vi "Test Sequence.vi"(0 "FeedBack Channel":string[](array[string])=["fgdgfvcbc", "vnfhgjkn", "21354682"], 1 "Test Name":string, 2 "Steps":T1(array[cluster]), 4 "WFGraph Refnum":refnum<vi>) -> (6 "Emergency":bool, 7 "Out":i32, 8 "Condition":bool)   [LabVIEW 2015]
uses:
  Galobal variable_TI.vi
  Project Setup/Globle Variable/GR_Servo.vi
  <vilib>/Instr/_visa.llb/VISA Configure Serial Port (Instr).vi
panel:
  out "error out 3":errorcluster
  out "Wait/Poll (ms)":u32
  out "Channels (Out)":i32[](array[numeric])
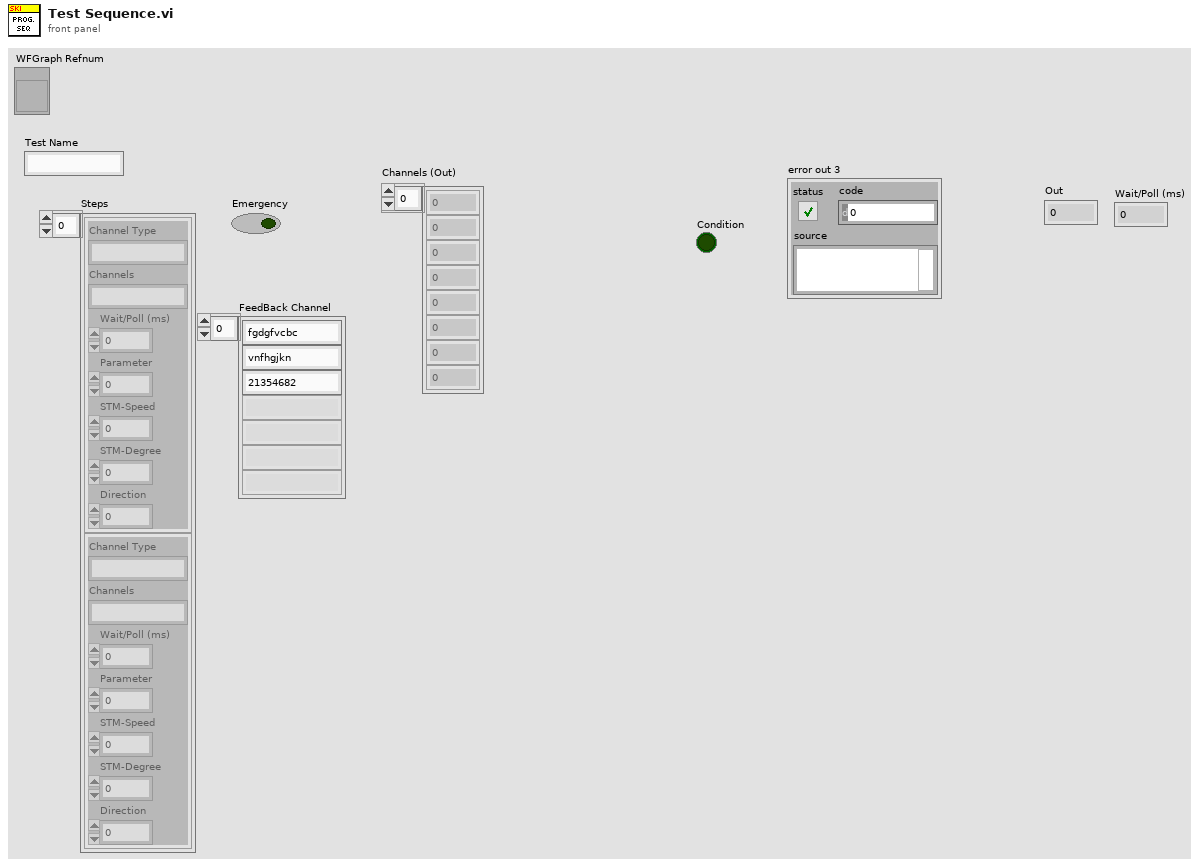
[diagram p1: front panel]
types:
  T1 = cluster{"Channel Type":string, "Channels":string, "Wait/Poll (ms)":u32, "Parameter":u8, "STM-Speed":i32, "STM-Degree":u32, "Direction":u8}[]
  T2 = cluster{"Emergency_1":bool, "Reset_2":bool, "Home _3":bool, "Air Pressure_4":bool, "Safety Sensor_5":bool, "Safety Sensor_6":bool, "Slide Servo Home RS 26":bool, "LVDT UP RS":bool, "Servo Fault 27":bool, "Pressing UP RS 31":bool, "40 Deg. Down Fixture Rs":bool}
  T3 = cluster{"MIC ":refnum<visa-resource-name>, "baud rate MIC ":u32, "LCD ":refnum<visa-resource-name>, "baud rate_LCD":u32}
  T4 = cluster{"Load Max(N)":dbl, "Load Min(N)":dbl, "Actuator1 max(mm)":dbl, "Actuator1min(mm)":dbl, "Actuator2 max(mm)":dbl, "Actuator2min(mm)":dbl, "Load Offset":dbl, "Model":string, "MIC Code":string}
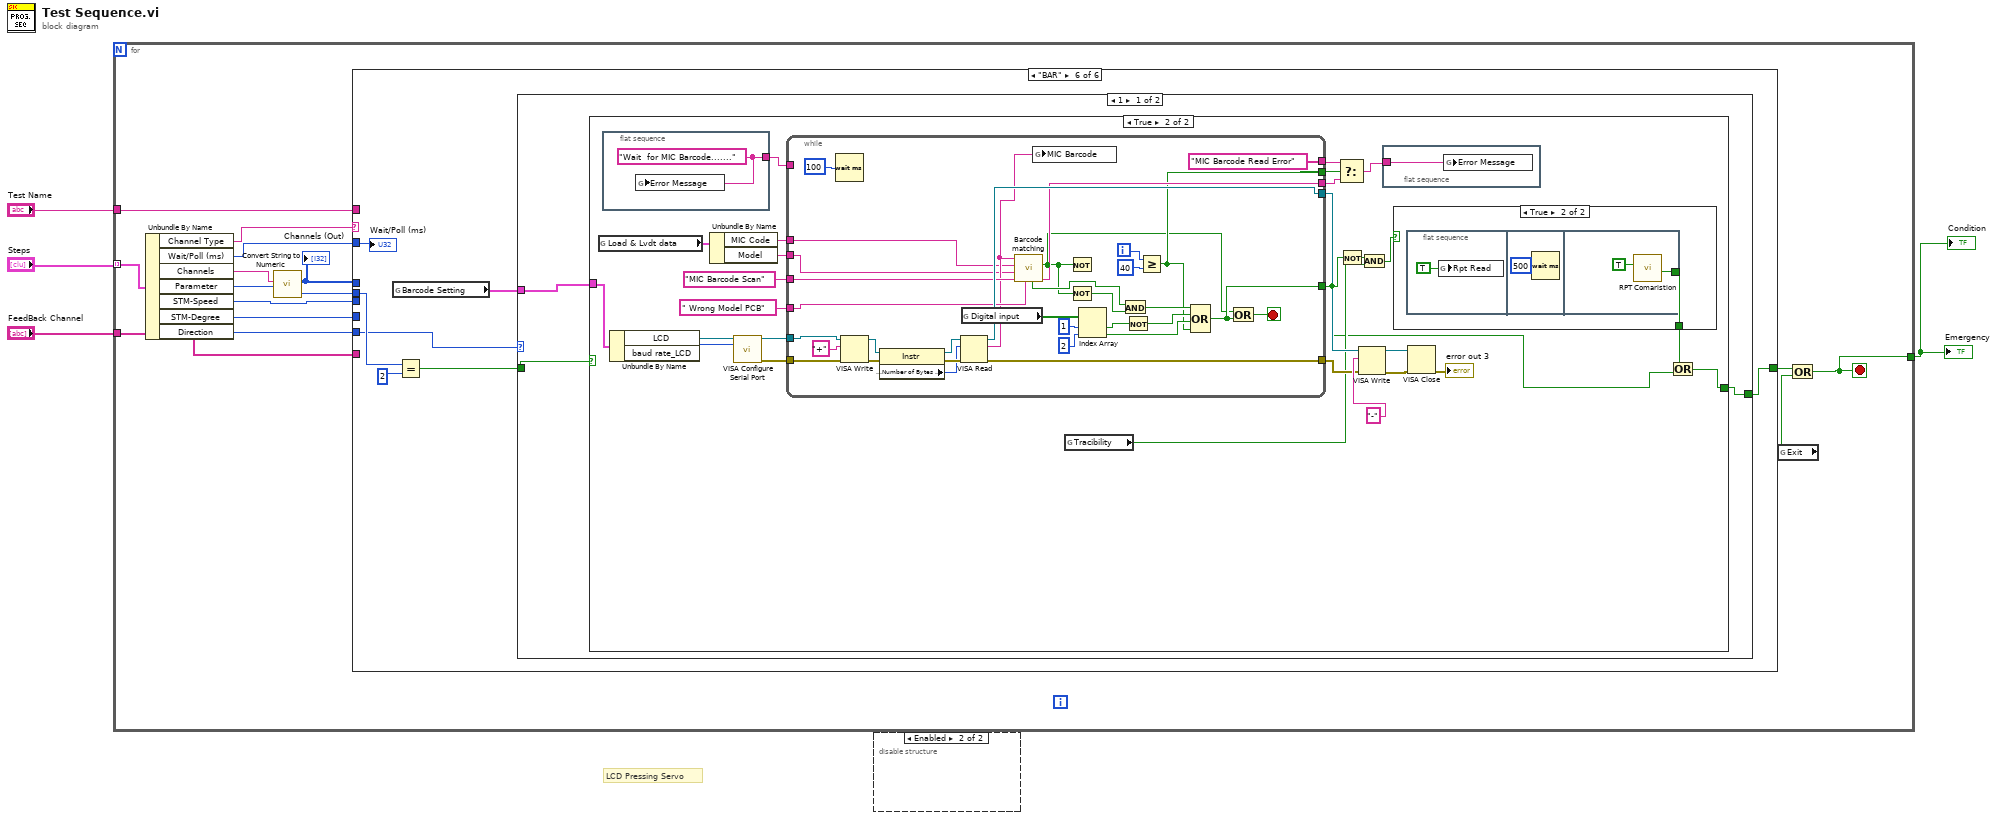
[diagram p0: block diagram]
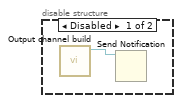
[diagram p2: hidden frame]
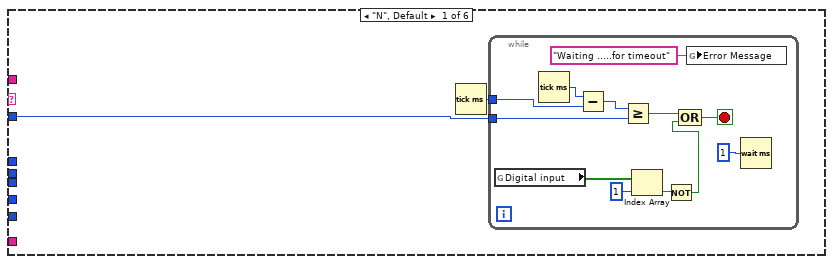
[diagram p3: hidden frame]
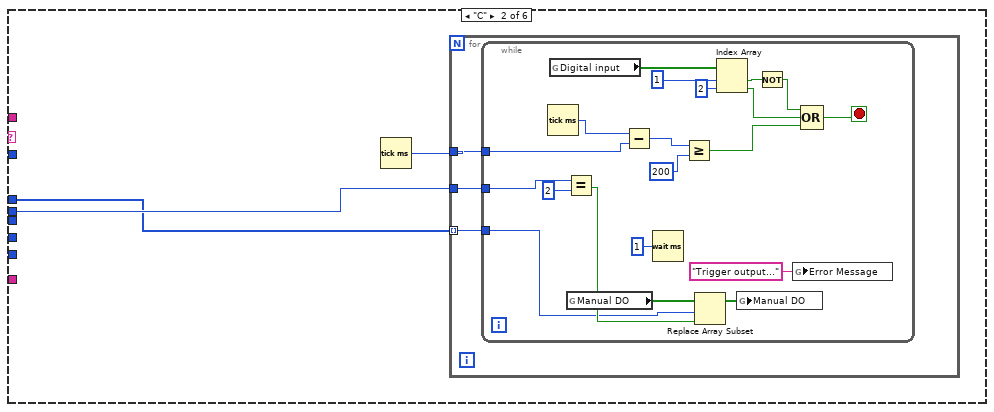
[diagram p4: hidden frame]
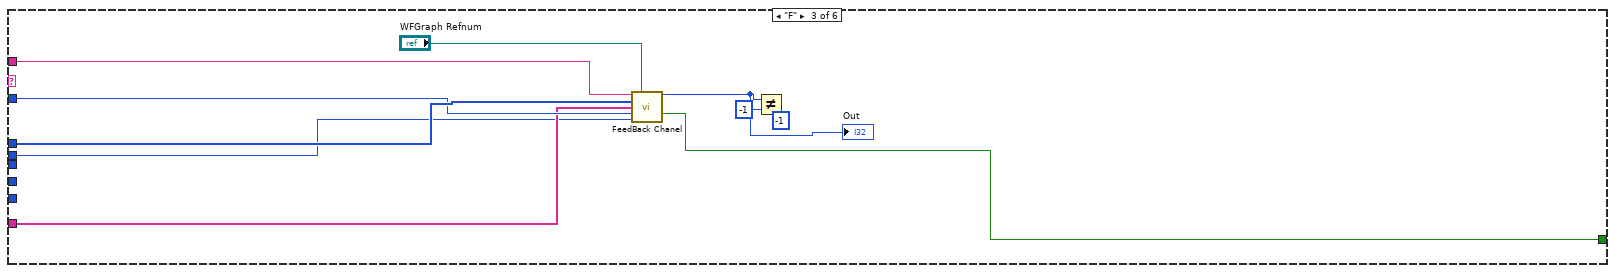
[diagram p5: hidden frame]
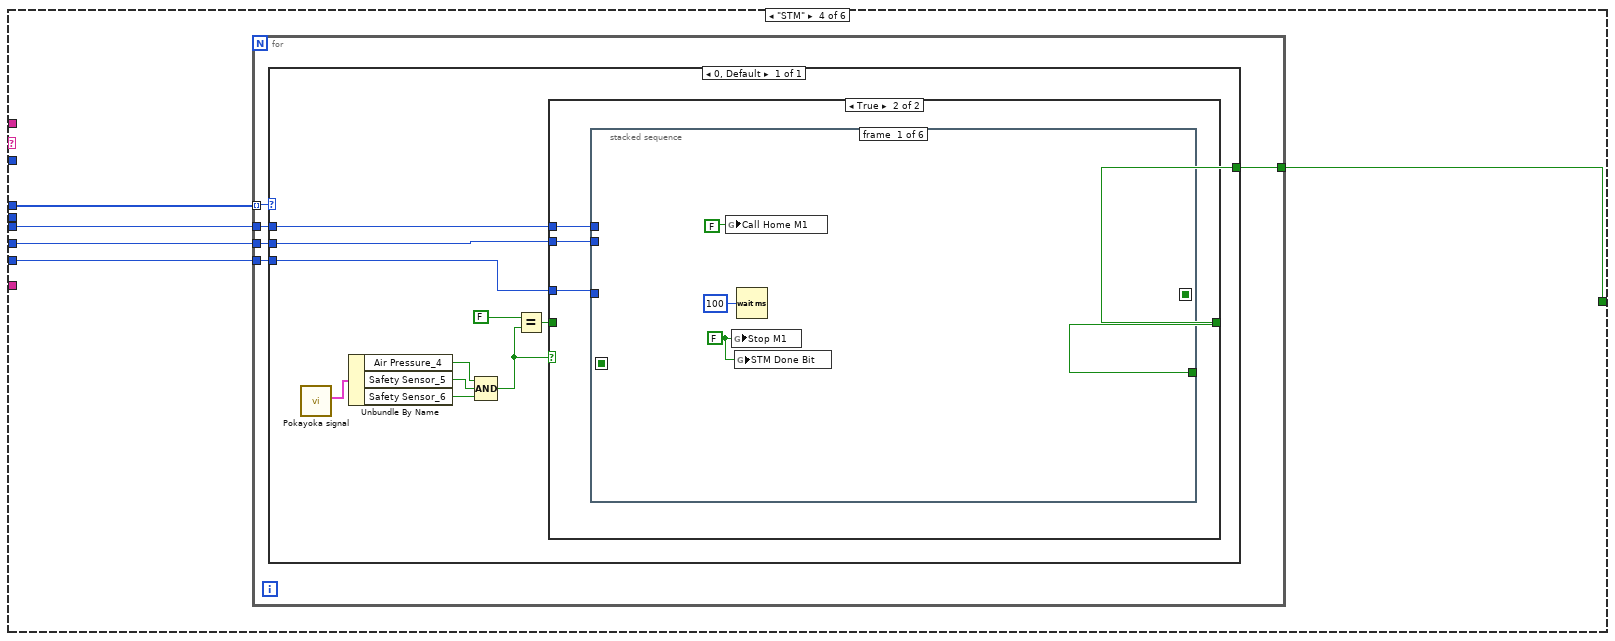
[diagram p6: hidden frame]
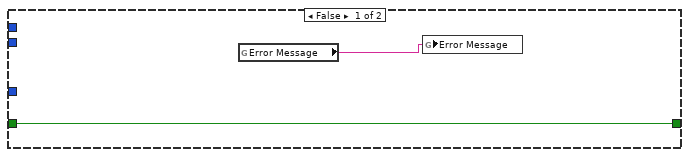
[diagram p7: hidden frame]
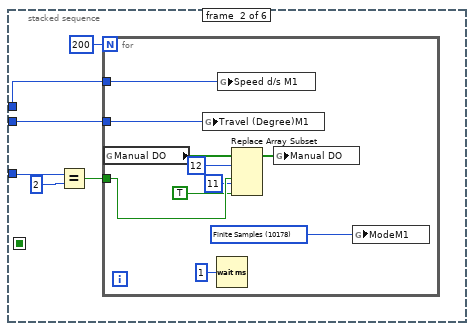
[diagram p8: hidden frame]
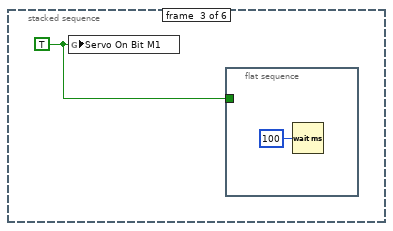
[diagram p9: hidden frame]
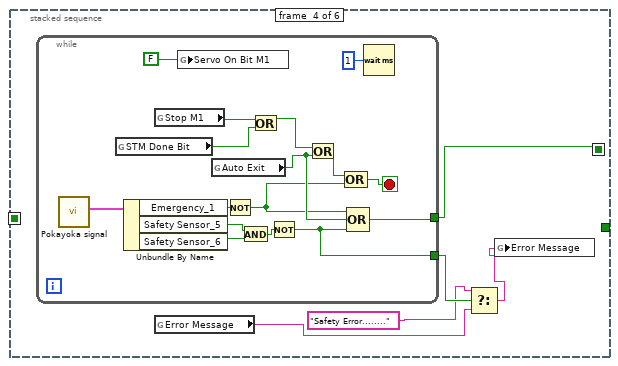
[diagram p10: hidden frame]
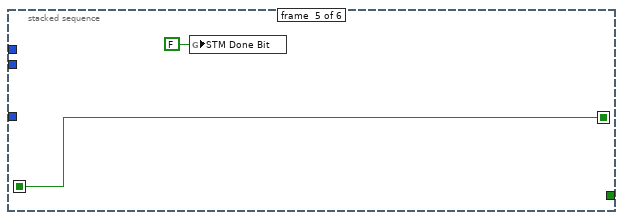
[diagram p11: hidden frame]
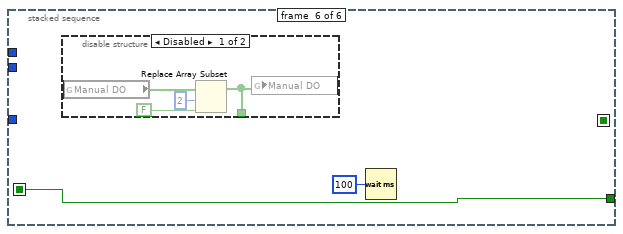
[diagram p12: hidden frame]
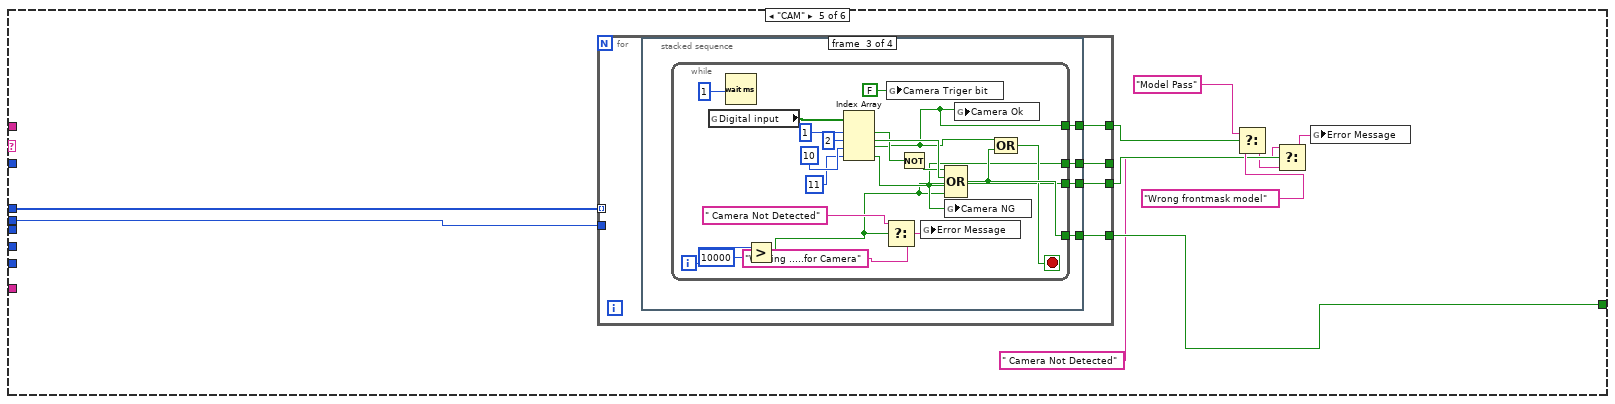
[diagram p14: hidden frame]
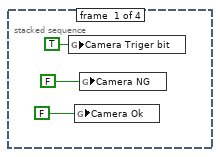
[diagram p15: hidden frame]
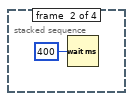
[diagram p16: hidden frame]
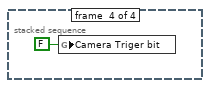
[diagram p17: hidden frame]
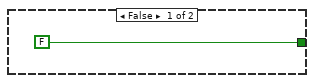
[diagram p18: hidden frame]
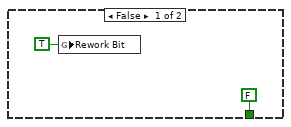
[diagram p19: hidden frame]
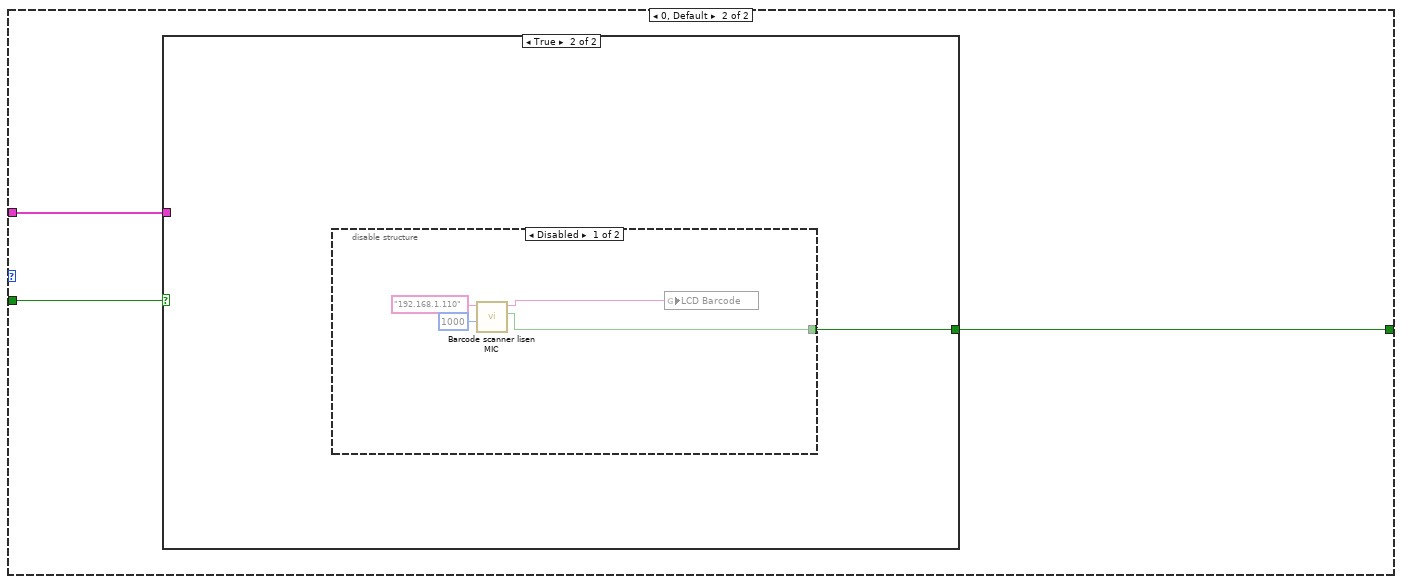
[diagram p20: hidden frame]
diagram:
  # "LCD Pressing Servo"
  n1 = for {
    tunnel: "Steps" -> [w18] mode=indexing
    tunnel: [w5] -> w1
    tunnel: "Test Name" -> [w13]
    tunnel: "FeedBack Channel" -> [w12]
    stop <- w5 stop-if-true
    n2 = Unbundle By Name(w18) -> ("Channel Type"=w17:string, "Wait/Poll (ms)"=w16:u32, "Channels"=w15:string, "Parameter"=w6:u8, "STM-Speed"=w8:i32, "STM-Degree"=w7:u32, "Direction"=w9:u8)
    n3 = call "Convert String to Numeric.vi"("Channels (A:B:C:D...) (In)"=w15) -> ("Channels (Out)"=w14:i32[])  [unwired: 9 in, 1 out]
    "Channels (Out)" <- w14
    n4 = case shown="\"BAR\"" w17 {
      tunnel: w16 -> [w19 _ w66 _ _ w194]
      tunnel: w14 -> [_ w33 w67 w72 w154 _]
      tunnel: w9 -> [_ _ _ w71 _ w188]
      tunnel: w13 -> [_ _ w65 _ _ _]
      tunnel: w12 -> [_ _ w64 _ _ _]
      tunnel: [_ _ w62 w68 w152 w189] -> w10
      tunnel: w8 -> [_ _ _ w70 _ _]
      tunnel: w7 -> [_ _ _ w69 _ _]
      tunnel: w6 -> [_ w35 w63 _ w153 w193]
      frame "N", Default {
        n5 = Tick Count (ms)() -> (millisecond timer value=w20:u32)
        n6 = while {
          tunnel: w20 -> [w31]
          tunnel: w19 -> [w26]
          stop <- w27 stop-if-true
          n7 = global read "Galobal variable_TI.vi" "Digital input"() -> (w25:bool[])
          n8 = Tick Count (ms)() -> (millisecond timer value=w32:u32)
          n9 = Subtract(x=w32, y=w31) -> (x-y=w30:u32)
          n10 = Greater Or Equal?(x=w30, y=w26) -> (x >= y?=w28:bool)
          n11 = Index Array(array=w25, index=1) -> (element=w23:bool)
          n12 = Not(x=w23) -> (.not. x?=w22:bool)
          n13 = Compound Arithmetic op=OR(w28, w22) -> (w27:bool)
          n14 = global write "GR_Servo.vi" "Error Message"("Waiting .....for timeout" ("Error Message")) -> ()
          n15 = Wait (ms)(milliseconds to wait=u32 1) -> ()  [unwired: 1 out]
        }
      }
      frame "C" {
        n16 = Tick Count (ms)() -> (millisecond timer value=w34:u32)
        n17 = for {
          tunnel: w33 -> [w37] mode=indexing
          tunnel: w35 -> [w38]
          tunnel: w34 -> [w36]
          n18 = while {
            tunnel: w38 -> [w58]
            tunnel: w37 -> [w52]
            tunnel: w36 -> [w50]
            stop <- w46 stop-if-true
            n19 = Tick Count (ms)() -> (millisecond timer value=w51:u32)
            n20 = global read "Galobal variable_TI.vi" "Digital input"() -> (w45:bool[])
            n21 = Equal?(x=w58, y=u8 2) -> (x = y?=w53:bool)
            n22 = global read "Galobal variable_TI.vi" "Manual DO"() -> (w54:bool[])
            n23 = Subtract(x=w51, y=w50) -> (x-y=w49:u32)
            n24 = Wait (ms)(milliseconds to wait=u32 1) -> ()  [unwired: 1 out]
            n25 = Greater Or Equal?(x=w49, y=u32 200) -> (x >= y?=w47:bool)
            n26 = Replace Array Subset(array=w54, new element=w53, index=w52) -> (w55:bool[])
            n27 = Index Array(array=w45, index #1=1 ("index"), index #2=2 ("index")) -> (element #1=w43:bool, element #2=w40:bool)
            n28 = global write "Galobal variable_TI.vi" "Manual DO"(w55) -> ()
            n29 = Not(x=w43) -> (.not. x?=w41:bool)
            n30 = global write "GR_Servo.vi" "Error Message"("Trigger output..." ("Error Message")) -> ()
            n31 = Compound Arithmetic op=OR(w41, w40, w47) -> (w46:bool)
          }
        }
      }
      frame "F" {
        (unwired) -1 ("Out")
        n32 = call "FeedBack Chanel.vi"("Test Name"=w65, "WFGraph Refnum"="WFGraph Refnum", "Channels (Int)"=w67, "FeedBack Channel"=w64, "Wait/Poll (ms)"=w66, "Parameter"=w63) -> ("Out"=w60:i32, "Fail"=w62:bool)  [unwired: 5 in, 3 out]
        "Out" <- w60
        n33 = Not Equal?(x=w60, y=-1) -> ()  [unwired: 1 out]
      }
      frame "STM" {
        n34 = for {
          tunnel: w72 -> [w77] mode=indexing
          tunnel: w71 -> [w76]
          tunnel: w70 -> [w75]
          tunnel: w69 -> [w74]
          tunnel: [w73] -> w68
          n35 = case shown="0, Default" w77 {
            tunnel: w76 -> [w86]
            tunnel: w75 -> [w88]
            tunnel: w74 -> [w87]
            tunnel: [w83] -> w73
            frame 0, Default {
              n36 = call "Pokayoka signal.vi"() -> ("output cluster"=w82:T2)  [unwired: 10 in, 1 out]
              n37 = Unbundle By Name(w82) -> ("Air Pressure_4"=w81:bool, "Safety Sensor_5"=w80:bool, "Safety Sensor_6"=w79:bool)
              n38 = Compound Arithmetic op=AND(w81, w80, w79) -> (w78:bool)
              n39 = Equal?(x=FALSE ("y"), y=w78) -> (x = y?=w84:bool)
              n40 = case shown="True" w78 {
                tunnel: w88 -> [_ w94]
                tunnel: w87 -> [_ w93]
                tunnel: w86 -> [_ w92]
                tunnel: [w90 w91] -> w83
                tunnel: w84 -> [w90 _]
                frame False {
                  n41 = global read "GR_Servo.vi" "Error Message"() -> (w89:string)
                  n42 = global write "GR_Servo.vi" "Error Message"(w89) -> ()
                }
                frame True {
                  n43 = stacked-sequence {
                    seq-local: [_ _ _ w120 _ _] -> [_ _ _ _ w137 _]
                    seq-local: [_ _ _ _ w137 _] -> [_ _ _ _ _ w139]
                    tunnel: w93 -> [_ w103 _ _ _ _]
                    tunnel: w92 -> [_ w101 _ _ _ _]
                    tunnel: w94 -> [_ w99 _ _ _ _]
                    tunnel: [_ _ _ _ _ w139] -> w91
                    frame #0 {
                      w95 = FALSE ("Stop M1")
                      n44 = global write "Galobal variable_TI.vi" "Call Home M1"(FALSE ("Call Home M2")) -> ()
                      n45 = global write "Galobal variable_TI.vi" "Stop M1"(w95) -> ()
                      n46 = global write "Galobal variable_TI.vi" "STM Done Bit"(w95) -> ()
                      n47 = Wait (ms)(milliseconds to wait=u32 100) -> ()  [unwired: 1 out]
                    }
                    frame #1 {
                      n48 = Equal?(x=w101, y=u8 2) -> (x = y?=w100:bool)
                      n49 = for {
                        N: 200 -> [_]
                        tunnel: w103 -> [w113]
                        tunnel: w100 -> [w111]
                        tunnel: w99 -> [w109]
                        w112 = 10178 items=["Finite Samples"=10178, "Continuous Samples"=10123, "Hardware Timed Single Point"=12522] ("ModeM1")
                        n50 = global read "Galobal variable_TI.vi" "Manual DO"() -> (w107:bool[])
                        n51 = global write "GR_Servo.vi" "Travel (Degree)M1"(w113) -> ()
                        n52 = Wait (ms)(milliseconds to wait=u32 1) -> ()  [unwired: 1 out]
                        n53 = global write "GR_Servo.vi" "Speed d/s M1"(w109) -> ()
                        n54 = Replace Array Subset(array=w107, new element #1=w111, index #1=12 ("index"), new element #2=TRUE ("new element/subarray"), index #2=11 ("index")) -> (w110:bool[])
                        n55 = global write "Galobal variable_TI.vi" "Manual DO"(w110) -> ()
                        n56 = global write "GR_Servo.vi" "ModeM1"(w112) -> ()
                      }
                    }
                    frame #2 {
                      w114 = TRUE ("Servo On Bit")
                      n57 = global write "GR_Servo.vi" "Servo On Bit M1"(w114) -> ()
                      n58 = flat-sequence {
                        tunnel: w114 -> [_]
                        frame #0 {
                          n59 = Wait (ms)(milliseconds to wait=u32 100) -> ()  [unwired: 1 out]
                        }
                      }
                    }
                    frame #3 {
                      n60 = while {
                        tunnel: [w126] -> w120
                        tunnel: [w121] -> w119
                        stop <- w129 stop-if-true
                        n61 = call "Pokayoka signal.vi"() -> ("output cluster"=w131:T2)  [unwired: 10 in, 1 out]
                        n62 = global read "Galobal variable_TI.vi" "STM Done Bit"() -> (w134:bool)
                        n63 = Unbundle By Name(w131) -> ("Emergency_1"=w128:bool, "Safety Sensor_5"=w124:bool, "Safety Sensor_6"=w123:bool)
                        n64 = global read "Galobal variable_TI.vi" "Stop M1"() -> (w135:bool)
                        n65 = global write "GR_Servo.vi" "Servo On Bit M1"(FALSE ("Servo On Bit")) -> ()
                        n66 = global read "Galobal variable_TI.vi" "Auto Exit"() -> (w127:bool)
                        n67 = Not(x=w128) -> (.not. x?=w125:bool)
                        n68 = And(x=w124, y=w123) -> (x .and. y?=w122:bool)
                        n69 = Or(x=w135, y=w134) -> (x .or. y?=w132:bool)
                        n70 = Not(x=w122) -> (.not. x?=w121:bool)
                        n71 = Or(x=w132, y=w127) -> (x .or. y?=w130:bool)
                        n72 = Compound Arithmetic op=OR(w130, w125) -> (w129:bool)
                        n73 = Compound Arithmetic op=OR(w125, w127, w121) -> (w126:bool)
                        n74 = Wait (ms)(milliseconds to wait=u32 1) -> ()  [unwired: 1 out]
                      }
                      n75 = global read "GR_Servo.vi" "Error Message"() -> (w116:string)
                      n76 = Select(t="Safety Error........" ("Error Message"), s=w119, f=w116) -> (s? t:f=w117:string)
                      n77 = global write "GR_Servo.vi" "Error Message"(w117) -> ()
                    }
                    frame #4 {
                      n78 = global write "Galobal variable_TI.vi" "STM Done Bit"(FALSE ("STM Done Bit LCD Pressing")) -> ()
                    }
                    frame #5 {
                      n79 = disable-structure shown="Disabled" {
                        disable-tunnel: [w141 _] -> _
                        frame Disabled {
                          n80 = global read "Galobal variable_TI.vi" "Manual DO"() -> (w144:bool[])
                          n81 = Replace Array Subset(array=w144, new element=FALSE ("new element/subarray"), index=2) -> (w141:bool[])
                          n82 = global write "Galobal variable_TI.vi" "Manual DO"(w141) -> ()
                        }
                        frame Enabled {
                        }
                      }
                      n83 = Wait (ms)(milliseconds to wait=u32 100) -> ()  [unwired: 1 out]
                    }
                  }
                }
              }
            }
          }
        }
      }
      frame "CAM" {
        n84 = for {
          tunnel: w154 -> [_] mode=indexing
          tunnel: w153 -> [_]
          tunnel: [w158] -> w152
          tunnel: [w157] -> w151
          tunnel: [w156] -> _
          tunnel: [w155] -> w148
          n85 = stacked-sequence {
            tunnel: [_ _ w166 _] -> w158
            tunnel: [_ _ w165 _] -> w157
            tunnel: [_ _ w164 _] -> w156
            tunnel: [_ _ w163 _] -> w155
            frame #0 {
              n86 = global write "Galobal variable_TI.vi" "Camera Triger bit"(TRUE ("Camera Triger bit")) -> ()
              n87 = global write "Galobal variable_TI.vi" "Camera Ok"(FALSE ("Camera Triger bit")) -> ()
              n88 = global write "Galobal variable_TI.vi" "Camera NG"(FALSE ("Camera Triger bit")) -> ()
            }
            frame #1 {
              n89 = Wait (ms)(milliseconds to wait=u32 400) -> ()  [unwired: 1 out]
            }
            frame #2 {
              n90 = while {
                tunnel: [w180] -> w166
                tunnel: [w170] -> w165
                tunnel: [w169] -> w164
                tunnel: [w168] -> w163
                i -> [w179]
                stop <- w174 stop-if-true
                n91 = global read "Galobal variable_TI.vi" "Digital input"() -> (w181:bool[])
                n92 = Wait (ms)(milliseconds to wait=u32 1) -> ()  [unwired: 1 out]
                n93 = Greater?(x=w179, y=10000) -> (0:w168:bool)
                n94 = Index Array(array=w181, index #1=1 ("index"), index #2=2 ("index"), index #3=10 ("index"), index #4=11 ("index")) -> (element #1=w184:bool, element #2=w186:bool, element #3=w170:bool, element #4=w169:bool)
                n95 = Select(t=" Camera Not Detected" ("Error Message"), s=w168, f="Waiting .....for Camera" ("Error Message")) -> (s? t:f=w175:string)
                n96 = global write "Galobal variable_TI.vi" "Camera Triger bit"(FALSE ("Camera Triger bit")) -> ()
                n97 = Not(x=w184) -> (.not. x?=w185:bool)
                n98 = global write "GR_Servo.vi" "Error Message"(w175) -> ()
                n99 = Compound Arithmetic op=OR(w185, w186, w169, w168) -> (w180:bool)
                n100 = global write "Galobal variable_TI.vi" "Camera NG"(w169) -> ()
                n101 = global write "Galobal variable_TI.vi" "Camera Ok"(w170) -> ()
                n102 = Compound Arithmetic op=OR(w170, w180) -> (w174:bool)
              }
            }
            frame #3 {
              n103 = global write "Galobal variable_TI.vi" "Camera Triger bit"(FALSE ("Camera Triger bit")) -> ()
            }
          }
        }
        n104 = Select(t="Model Pass", s=w151, f="Wrong frontmask model") -> (s? t:f=w146:string)
        n105 = Select(t=" Camera Not Detected" ("Error Message"), s=w148, f=w146) -> (s? t:f=w145:string)
        n106 = global write "GR_Servo.vi" "Error Message"(w145) -> ()
      }
      frame "BAR" {
        n107 = global read "Galobal variable_TI.vi" "Barcode Setting"() -> (w190:T3)
        n108 = Equal?(x=w193, y=u8 2) -> (x = y?=w191:bool)
        n109 = case shown="1" w188 {
          tunnel: w191 -> [w197 w270]
          tunnel: w190 -> [w196 w269]
          tunnel: [w195 w268] -> w189
          frame 1 {
            n110 = case shown="True" w197 {
              tunnel: w196 -> [_ w211]
              tunnel: [FALSE w199] -> w195
              frame False {
              }
              frame True {
                n111 = global read "Galobal variable_TI.vi" "Load & Lvdt data"() -> (w205:T4)
                n112 = flat-sequence {
                  tunnel: [w234] -> w221
                  frame #0 {
                    w234 = "Wait  for MIC Barcode......."
                    n113 = global write "GR_Servo.vi" "Error Message"(w234) -> ()
                  }
                }
                n114 = Unbundle By Name(w211) -> ("LCD"=w213:refnum<visa-resource-name>, "baud rate_LCD"=w214:u32)
                n115 = Unbundle By Name(w205) -> ("MIC Code"=w217:string, "Model"=w218:string)
                n116 = call-poly "VISA Configure Serial Port"("VISA resource name"=w213, "baud rate (9600)"=w214) -> ("VISA resource name out"=w215:refnum<visa-resource-name>, "error out"=w216:errorcluster)  [unwired: 12 in]
                n117 = while {
                  tunnel: w215 -> [w252]
                  tunnel: w216 -> [w251]
                  tunnel: [w264] -> w209
                  tunnel: [w263] -> w208
                  tunnel: [w247] -> w201
                  tunnel: w217 -> [w236]
                  tunnel: w218 -> [w237]
                  tunnel: "MIC Barcode Scan" ("TFT BARCODE SCANE") -> [w255]
                  tunnel: " Wrong Model PCB" ("TFT WORNG SCANE") -> [w254]
                  tunnel: w221 -> [_]
                  tunnel: [w246] -> w224
                  tunnel: [w240] -> w222
                  tunnel: ["MIC Barcode Read Error"] -> w223
                  i -> [w241]
                  stop <- w248 stop-if-true
                  n118 = Wait (ms)(milliseconds to wait=u32 100) -> ()  [unwired: 1 out]
                  n119 = VISA Write(VISA resource name=w252, write buffer="+", error in (no error)=w251) -> (VISA resource name out=w250:refnum<visa-resource-name>, error out=w249:errorcluster)  [unwired: 1 out]
                  n120 = property class="Instr"(reference=w250, error in=w249) -> (reference out=w267:refnum<visa-resource-name>, error out=w266:errorcluster, "Serial Settings:Number of Bytes at Serial Port"=w265:u32)
                  n121 = VISA Read(VISA resource name=w267, byte count=w265, error in (no error)=w266) -> (VISA resource name out=w264:refnum<visa-resource-name>, read buffer=w238:string, error out=w263:errorcluster)  [unwired: 1 out]
                  n122 = global read "Galobal variable_TI.vi" "Digital input"() -> (w262:bool[])
                  n123 = call "Barcode matching.vi"("TFT WORNG SCANE"=w254, "TFT BARCODE SCANE"=w255, "Model"=w237, "TFT Code"=w236, "Serial data"=w238) -> ("Error"=w246:string, "result/trigger"=w235:bool, "Read bit"=w244:bool)  [unwired: 2 in, 2 out]
                  n124 = global write "Galobal variable_TI.vi" "MIC Barcode"(w238) -> ()
                  n125 = Not(x=w235) -> ()  [unwired: 1 out]
                  n126 = Not(x=w235) -> (.not. x?=w245:bool)
                  n127 = Index Array(array=w262, index #1=1 ("index"), index #2=2 ("index")) -> (element #1=w259:bool, element #2=w257:bool)
                  n128 = And(x=w244, y=w245) -> (x .and. y?=w243:bool)
                  n129 = Not(x=w259) -> (.not. x?=w258:bool)
                  n130 = Greater Or Equal?(x=w241, y=40) -> (x >= y?=w240:bool)
                  n131 = Compound Arithmetic op=OR(w243, w258, w257, w240) -> (w247:bool)
                  n132 = Compound Arithmetic op=OR(w235, w247) -> (w248:bool)
                }
                n133 = global read "Galobal variable_TI.vi" "Tracibility"() -> (w204:bool)
                n134 = Select(t=w223, s=w222, f=w224) -> (s? t:f=w225:string)
                n135 = Not(x=w201) -> (.not. x?=w202:bool)
                n136 = VISA Write(VISA resource name=w209, write buffer="-", error in (no error)=w208) -> (VISA resource name out=w207:refnum<visa-resource-name>, error out=w206:errorcluster)  [unwired: 1 out]
                n137 = And(x=w202, y=w204) -> (x .and. y?=w203:bool)
                n138 = flat-sequence {
                  tunnel: w225 -> [w233]
                  frame #0 {
                    n139 = global write "GR_Servo.vi" "Error Message"(w233) -> ()
                  }
                }
                n140 = case shown="True" w203 {
                  tunnel: [FALSE ("Fail") w228] -> w200
                  frame False {
                    n141 = global write "Galobal variable_TI.vi" "Rework Bit"(TRUE ("Rework bit")) -> ()
                  }
                  frame True {
                    n142 = flat-sequence {
                      tunnel: [w231] -> w228
                      frame #0 {
                        n143 = global write "Galobal variable_TI.vi" "Rpt Read"(TRUE ("Rpt Read")) -> ()
                      }
                      frame #1 {
                        n144 = Wait (ms)(milliseconds to wait=u32 500) -> ()  [unwired: 1 out]
                      }
                      frame #2 {
                        n145 = call "RPT Comaristion.vi"("True"=TRUE) -> ("Fail"=w231:bool)  [unwired: 10 in]
                      }
                    }
                  }
                }
                n146 = VISA Close(VISA resource name=w207, error in (no error)=w206) -> (error out=→"error out 3":errorcluster)
                n147 = Or(x=w200, y=w201) -> (x .or. y?=w199:bool)
              }
            }
          }
          frame 0, Default {
            n148 = case shown="True" w270 {
              tunnel: w269 -> [_ _]
              tunnel: [FALSE w272] -> w268
              frame False {
                # "barcode bypass"
              }
              frame True {
                n149 = disable-structure shown="Disabled" {
                  disable-tunnel: [w273 _] -> w272
                  frame Disabled {
                    n150 = call "Barcode scanner lisen MIC.vi"("port"=u16 1000, "service name"="192.168.1.110") -> ("Exit"=w273:bool, "data out"=w274:string)  [unwired: 7 in, 1 out]
                    n151 = global write "Galobal variable_TI.vi" "LCD Barcode"(w274) -> ()
                  }
                  frame Enabled {
                  }
                }
              }
            }
          }
        }
        "Wait/Poll (ms)" <- w194
      }
    }
    n152 = global read "Galobal variable_TI.vi" "Exit"() -> (w11:bool)
    n153 = Compound Arithmetic op=OR(w10, w11) -> (w5:bool)
  }
  "Emergency" <- w1
  "Condition" <- w1
  n154 = disable-structure shown="Enabled" {
    frame Disabled {
      n155 = call "Output channel build.vi"() -> ("Output channel"=w277:refnum<notifier>)  [unwired: 11 in]
      n156 = Send Notification(notifier=w277) -> ()  [unwired: 2 in, 2 out]
    }
    frame Enabled {
    }
  }
